vi "main.vi"() -> ()   [LabVIEW 2017]
uses:
  <vilib>/Platform/TimedLoop/XDataNode/timing_clust.ctl
  <vilib>/Platform/TimedLoop/XDataNode/nitl_modes.ctl
  <vilib>/Platform/TimedLoop/XDataNode/wakeup.ctl
  <vilib>/Instr/_visa.llb/VISA Configure Serial Port (Instr).vi
  <vilib>/Platform/TimedLoop/XDataNode/XDataNode.xnode
  <vilib>/Platform/TimedLoop/XDataNode/XDNodeRunTimeDep.lvlib
panel:
  out "TX":dbl
  out "RX":dbl
  in  "连接":bool
  out "串口状态":bool
  in  "波特率":u16(ring) items=["9600", "115200"]
  in  "端口":string(combo)
  in  "界面切换":enum32{"选项卡 1", "调试助手"}(tab)
  in  "清空波形":bool
  out "DA1计算值":dbl
  out "DA0计算值":dbl
  in  "清空曲线":bool
  in  "持续时间":string
  in  "系统时间":string
  in  "发送波形":bool
  out "波形图":dbl[](graph)
  in  "波形选择":enum32{"斜坡", "正弦", "PWM波", "直流", "抛物线", ""}(tab)
  out "斜率k":dbl format="%#.2g"
  in  "通道D":enum16{"DA0", "DA1", "DA01", ""}(ring) caption="通道"
  in  "截距":dbl(slide) min=-5.0 max=5.0 step=0.01 scale=-4.0..4.0
  in  "斜率角":dbl(slide) step=0.01 scale=0.0..180.0
  in  "极值":dbl(slide) min=-5.0 max=5.0 step=0.01 scale=-4.0..4.0
  out "正弦频率":dbl caption="频率 f" format="%#.2g"
  in  "偏距":dbl(slide) min=-5.0 max=5.0 step=0.01 scale=-4.0..4.0
  in  "初相":dbl(slide) min=-6.5 max=6.5 step=0.01 scale=-7.0..7.0
  in  "振幅":dbl(slide) min=0.0 max=5.0 step=0.01 scale=0.0..4.0
  in  "正弦角频率":dbl(slide) caption="角频率" min=0.0 max=100.0 step=0.01 scale=0.0..65.0
  in  "通道S":enum16{"DA0", "DA1", "DA01", ""}(ring) caption="通道"
  in  "通道P":enum16{"DA0", "DA1", "DA01", ""}(ring) caption="通道"
  in  "占空比":dbl(slide) min=0.0 max=1.0 step=0.01 scale=0.0..1.0
  in  "PWM波频率":dbl(slide) caption="频率" min=0.0 max=100.0 step=0.01 scale=0.0..10.0
  in  "低电压":dbl(slide) min=-5.0 max=5.0 step=0.01 scale=-4.0..4.0
  in  "高电压":dbl(slide) min=-5.0 max=5.0 step=0.01 scale=-4.0..4.0
  in  "DA0":dbl(slide) min=-5.0 max=5.0 step=0.01 scale=-4.0..4.0
  in  "DA1":dbl(slide) min=-5.0 max=5.0 step=0.01 scale=-4.0..4.0
  in  "板子选择":bool
  in  "换行":bool
  in  "发送区":string
  in  "send":bool
  in  "清空计数":bool
  in  "清空接收区":bool
  out "接收区":string
  # "y=kt+b"
  # "y=Asin(ωt+φ)+k"
  # "此页面无需点击“发送波形”按钮"
  # "y=k/(a*t+b)"
  # "y=kln(a)+b"
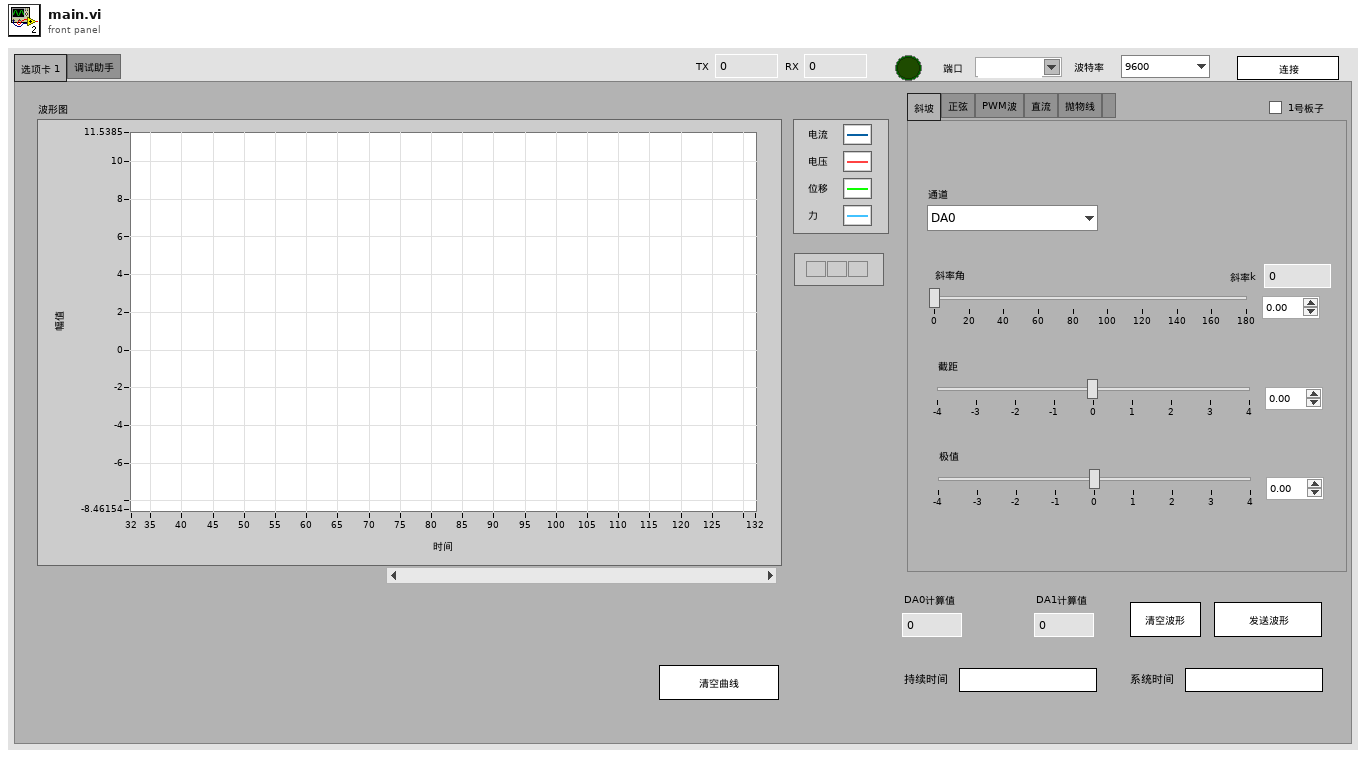
[diagram p1: front panel]
types:
  T1 = typedef "XDNodeRunTimeDep.lvlib/timing_clust.ctl" = cluster{"Expected End [f-1]":u64, "Actual End [f-1]":u64, "Finished Late? [f-1]":bool, "Expected End [i-1]":u64, "Actual End [i-1]":u64, "Finished Late? [i-1]":bool, "Expected Start [i]":u64, "Actual Start [i]":u64, "Expected Start [f]":u64, "Actual Start [f]":u64, "Source Name":string, "Structure Name":string, "Period":i64, "Deadline":i64, "Offset":i64, "Start":i64, "Priority":i32, "Timeout":i32, "Mode":T2, "Wakeup Reason":T3, "Error":errorcluster, "Source Type":string, "Secondary Source Type":string, "Global End Time":u64, "Global Start Time":u64, "Frame Duration":u64, "Iteration Duration":u64, "Assigned CPU":i32, "I/O Scan Engine Mode":u32}
  T2 = typedef "XDNodeRunTimeDep.lvlib/nitl_modes.ctl" = enum32{"No Change", "Process missed periods, maintain original phase", "Discard missed periods, maintain original phase", "Process missed periods, ignore original phase", "Discard missed periods, ignore original phase"}
  T3 = typedef "XDNodeRunTimeDep.lvlib/wakeup.ctl" = enum32{"Normal", "Aborted", "Asynchronous wakeup", "Timing source error", "Timed loop error", "Timeout"}
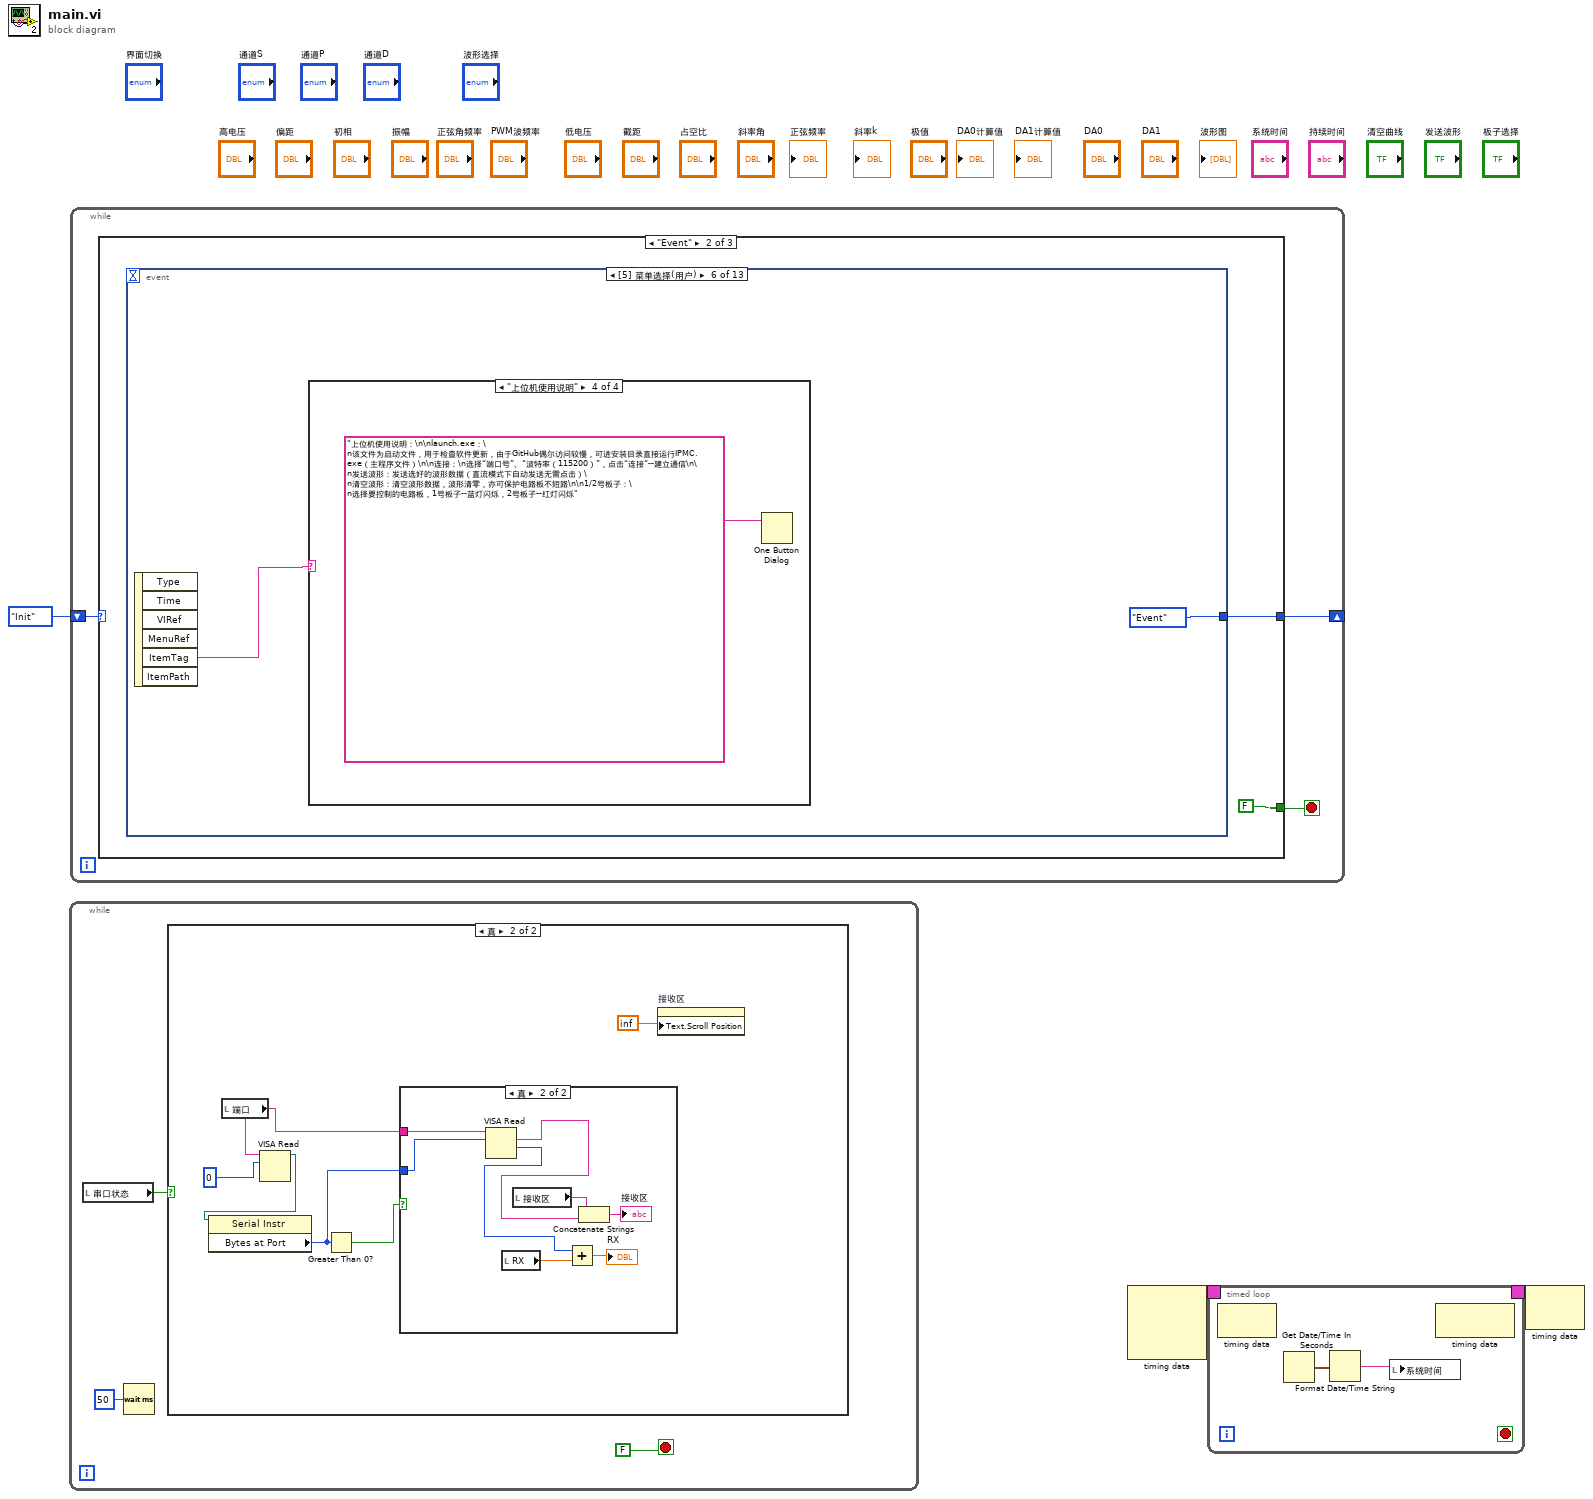
[diagram p0: block diagram]
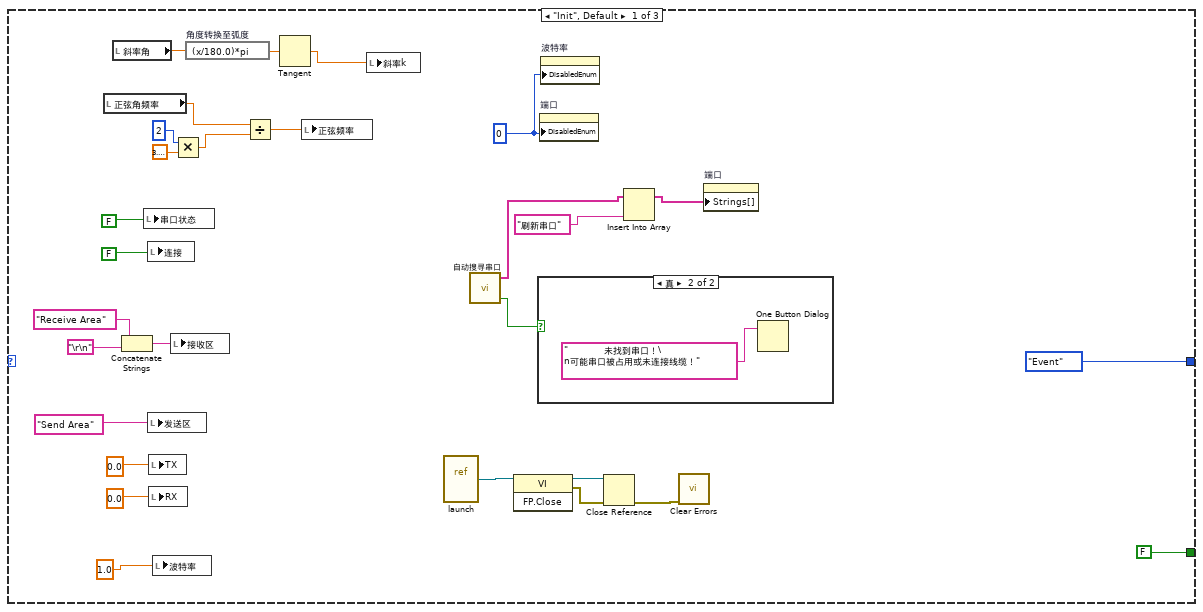
[diagram p4: hidden frame]
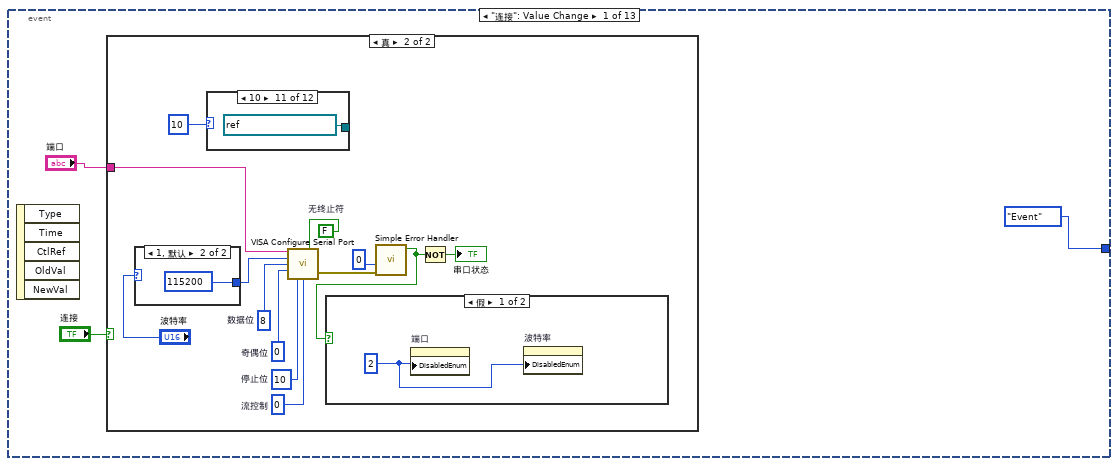
[diagram p6: hidden frame]
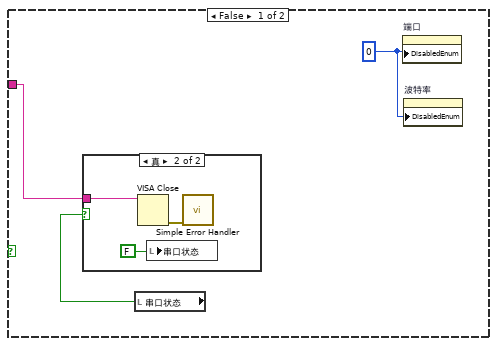
[diagram p7: hidden frame]
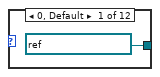
[diagram p9: hidden frame]
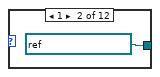
[diagram p10: hidden frame]
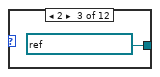
[diagram p11: hidden frame]
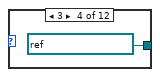
[diagram p12: hidden frame]
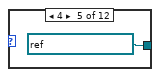
[diagram p13: hidden frame]
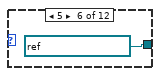
[diagram p14: hidden frame]
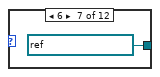
[diagram p15: hidden frame]
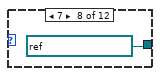
[diagram p16: hidden frame]
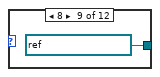
[diagram p17: hidden frame]
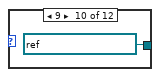
[diagram p18: hidden frame]
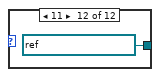
[diagram p19: hidden frame]
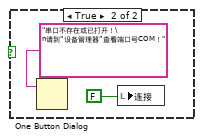
[diagram p20: hidden frame]
diagram:
  n1 = while {
    stop <- FALSE stop-if-true
    n2 = local read "串口状态"() -> (w6:bool)
    n3 = Wait (ms)(milliseconds to wait=u32 50 ("等待时间（毫秒）")) -> ()  [unwired: 1 out]
    n4 = case shown="真" w6 {
      frame False {
      }
      frame True {
        n5 = local read "端口"() -> (w10:string)
        n6 = VISA Read(VISA resource name=w10, byte count=0) -> (VISA resource name out=w9:refnum<visa-resource-name>)  [unwired: 1 in, 3 out]
        n7 = property class="Serial Instr"(reference=w9) -> ("Bytes at Port"=w7:u32)  [unwired: 1 in, 2 out]
        n8 = Greater Than 0?(x=w7) -> (x > 0?=w8:bool)
        n9 = case shown="真" w8 {
          tunnel: w10 -> [_ w14]
          tunnel: w7 -> [_ w13]
          frame False {
          }
          frame True {
            n10 = VISA Read(VISA resource name=w14, byte count=w13) -> (read buffer=w20:string, return count=w15:u32)  [unwired: 1 in, 2 out]
            n11 = local read "RX"() -> (w17:dbl)
            n12 = local read "接收区"() -> (w18:string)
            n13 = Add(x=w15, y=w17) -> (x+y=→"RX":dbl)
            n14 = Concatenate Strings(w18, w20) -> (→"接收区":string)
          }
        }
        n15 = property on="接收区" class="Str"("Text.Scroll Position"=inf) -> ()  [unwired: 2 in, 2 out]
      }
    }
  }
  n16 = while {
    shift-right: [w22] -> _
    shift-left: enum16{"Init", "Event", "Exit"}."Init" -> [w23]
    stop <- w21 stop-if-true
    n17 = case shown="\"Event\"" w23 {
      tunnel: [FALSE FALSE TRUE] -> w21
      tunnel: [enum16{"Init", "Event", "Exit"}."Event" w53 enum16{"Init", "Event", "Exit"}."Exit"] -> w22
      frame "Init", Default {
        w32 = 0
        n18 = local read "正弦角频率"() -> (w39:dbl)
        n19 = local read "斜率角"() -> (w43:dbl)
        n20 = Concatenate Strings("Receive Area", "\r\n") -> (w33:string)
        n21 = local write "串口状态"(FALSE) -> ()
        n22 = local write "连接"(FALSE) -> ()
        n23 = local write "发送区"("Send Area" ("发送区")) -> ()
        n24 = local write "TX"(0.0 ("TX")) -> ()
        n25 = local write "RX"(0.0 ("RX")) -> ()
        n26 = local write "波特率"(1.0 ("RX")) -> ()
        n27 = local write "接收区"(w33) -> ()
        n28 = Multiply(x=2, y=3.141592653589793) -> (x*y=w38:dbl)
        n29 = expression code="(x/180.0)*pi" "角度转换至弧度"(w43) -> (w44:dbl)
        n30 = Divide(x=w39, y=w38) -> (x/y=w40:dbl)
        n31 = Tangent(1:w44) -> (0:w37:dbl)
        n32 = local write "正弦频率"(w40) -> ()
        n33 = local write "斜率k"(w37) -> ()
        n34 = vi-ref "launch.vi"() -> (w27:refnum<vi>)
        n35 = call "自动搜寻串口.vi"() -> ("找到的串口"=w30:string[], "有错误?"=w31:bool)  [unwired: 6 in, 1 out]
        n36 = invoke class="VI" method="FP.Close"(reference=w27) -> (reference out=w26:refnum<vi>, error out=w25:errorcluster)  [unwired: 2 in, 1 out]
        n37 = case shown="真" w31 {
          frame False {
          }
          frame True {
            n38 = One Button Dialog(message="            未找到串口！\n可能串口被占用或未连接线缆！") -> ()  [unwired: 1 in, 1 out]
          }
        }
        n39 = property on="端口" class="CmbBox"("DisabledEnum"=w32) -> ()  [unwired: 2 in, 2 out]
        n40 = property on="波特率" class="Ring (严格)"("DisabledEnum"=w32) -> ()  [unwired: 2 in, 2 out]
        n41 = Close Reference(reference=w26, error in (no error)=w25) -> (error out=w24:errorcluster)
        n42 = Insert Into Array(array=w30, new element="刷新串口") -> (w28:string[])  [unwired: 1 in]
        n43 = call <vilib>:"Clear Errors.vi"("error in (no error)"=w24) -> ()  [unwired: 5 in, 2 out]
        n44 = property on="端口" class="CmbBox"("Strings[]"=w28) -> ()  [unwired: 2 in, 2 out]
      }
      frame "Event" {
        n45 = event shown="[5] 菜单选择(用户)" {
          selector: _ -> [_ _ _ _ _ _ _ _ _ _ _ _ _]
          dyn-events: _ -> [_ _ _ _ _ _ _ _ _ _ _ _ _]
          timeout: _ -> [_ _ _ _ _ _ _ _ _ _ _ _ _]
          tunnel: [enum16{"Init", "Event", "Exit"}."Event" _ enum16{"Init", "Event", "Exit"}."Event" enum16{"Init", "Event", "Exit"}."Event" enum16{"Init", "Event", "Exit"}."Event" enum16{"Init", "Event", "Exit"}."Event" enum16{"Init", "Event", "Exit"}."Event" enum16{"Init", "Event", "Exit"}."Event" enum16{"Init", "Event", "Exit"}."Event" enum16{"Init", "Event", "Exit"}."Event" enum16{"Init", "Event", "Exit"}."Event" enum16{"Init", "Event", "Exit"}."Event" enum16{"Init", "Event", "Exit"}."Event"] -> w53
          event "连接": Value Change {
            n46 = event-data() -> ()  [unwired: 1 in, 5 out]
            n47 = case shown="真" "连接" {
              tunnel: "端口" -> [w59 w64]
              frame False {
                w58 = 0
                n48 = local read "串口状态"() -> (w60:bool)
                n49 = case shown="真" w60 {
                  tunnel: w59 -> [_ w61]
                  frame False {
                  }
                  frame True {
                    n50 = VISA Close(VISA resource name=w61) -> (error out=w63:errorcluster)  [unwired: 1 in]
                    n51 = local write "串口状态"(FALSE) -> ()
                    n52 = call <vilib>:"Simple Error Handler.vi"("error in (no error)"=w63) -> ()  [unwired: 4 in, 5 out]
                  }
                }
                n53 = property on="端口" class="CmbBox"("DisabledEnum"=w58) -> ()  [unwired: 2 in, 2 out]
                n54 = property on="波特率" class="Ring (严格)"("DisabledEnum"=w58) -> ()  [unwired: 2 in, 2 out]
              }
              frame True {
                w67 = FALSE  # 无终止符
                w74 = u16 0  # 流控制
                w73 = u16 10  # 停止位
                w72 = u8 0  # 奇偶位
                w71 = u16 8  # 数据位
                n55 = case shown="1, 默认" "波特率" {
                  tunnel: [u32 9600 u32 115200] -> w70
                  frame 0 {
                  }
                  frame 1, Default {
                  }
                }
                n56 = case shown="10" 10 {
                  tunnel: [refnum<visa-resource-name> "ASRL1::INSTR" ("VISA resource name") refnum<visa-resource-name> "ASRL2::INSTR" ("VISA resource name") refnum<visa-resource-name> "ASRL3::INSTR" ("VISA resource name") refnum<visa-resource-name> "ASRL4::INSTR" ("VISA resource name") refnum<visa-resource-name> "ASRL5::INSTR" ("VISA resource name") refnum<visa-resource-name> "ASRL6::INSTR" ("VISA resource name") refnum<visa-resource-name> "ASRL7::INSTR" ("VISA resource name") refnum<visa-resource-name> "ASRL8::INSTR" ("VISA resource name") refnum<visa-resource-name> "ASRL9::INSTR" ("VISA resource name") refnum<visa-resource-name> "ASRL10::INSTR" ("VISA resource name") refnum<visa-resource-name> "ASRL11::INSTR" ("VISA resource name") refnum<visa-resource-name> "ASRL12::INSTR" ("VISA resource name")] -> _
                  frame 0, Default {
                  }
                  frame 1 {
                  }
                  frame 2 {
                  }
                  frame 3 {
                  }
                  frame 4 {
                  }
                  frame 5 {
                  }
                  frame 6 {
                  }
                  frame 7 {
                  }
                  frame 8 {
                  }
                  frame 9 {
                  }
                  frame 10 {
                  }
                  frame 11 {
                  }
                }
                n57 = call-poly "VISA Configure Serial Port"("VISA resource name"=w64, "Enable Termination\nChar (T)"=w67, "baud rate (9600)"=w70, "data bits (8)"=w71, "parity (0:none)"=w72, "stop bits (10: 1 bit)"=w73, "flow control (0:none)"=w74) -> ("error out"=w75:errorcluster)  [unwired: 7 in, 1 out]
                n58 = call <vilib>:"Simple Error Handler.vi"("type of dialog (OK msg:1)"=0, "error in (no error)"=w75) -> ("error?"=w68:bool)  [unwired: 3 in, 4 out]
                n59 = case shown="假" w68 {
                  frame False {
                    w89 = 2
                    n60 = property on="端口" class="CmbBox"("DisabledEnum"=w89) -> ()  [unwired: 2 in, 2 out]
                    n61 = property on="波特率" class="Ring (严格)"("DisabledEnum"=w89) -> ()  [unwired: 2 in, 2 out]
                  }
                  frame True {
                    n62 = One Button Dialog(message="串口不存在或已打开！\n请到“设备管理器”查看端口号COM！") -> ()  [unwired: 1 in, 1 out]
                    n63 = local write "连接"(FALSE) -> ()
                  }
                }
                n64 = Not(x=w68) -> (.not. x?=→"串口状态":bool)
              }
            }
          }
          event "端口": Value Change {
            n65 = event-data() -> ("NewVal"=w96:string)  [unwired: 1 in, 5 out]
            n66 = Equal?(x=w96, y="刷新串口") -> (x = y?=w94:bool)
            n67 = case shown="真" w94 {
              frame False {
              }
              frame True {
                n68 = call "自动搜寻串口.vi"() -> ("找到的串口"=w98:string[], "有错误?"=w100:bool)  [unwired: 6 in, 1 out]
                n69 = case shown="真" w100 {
                  frame False {
                  }
                  frame True {
                    n70 = One Button Dialog(message="            未找到串口！\n可能串口被占用或未连接线缆！") -> ()  [unwired: 1 in, 1 out]
                  }
                }
                n71 = Insert Into Array(array=w98, new element="刷新串口") -> (w97:string[])  [unwired: 1 in]
                n72 = property on="端口" class="CmbBox"("Strings[]"=w97) -> ()  [unwired: 2 in, 2 out]
              }
            }
          }
          event "send": Mouse Down {
            n73 = event-data() -> ()  [unwired: 1 in, 7 out]
            n74 = local read "串口状态"() -> (w103:bool)
            n75 = case shown="真" w103 {
              frame False {
              }
              frame True {
                n76 = local read "端口"() -> (w104:string)
                n77 = case shown="真" "换行" {
                  tunnel: [_ "\r"] -> w112
                  tunnel: [_ "\n"] -> w111
                  frame False {
                  }
                  frame True {
                  }
                }
                n78 = Concatenate Strings("发送区", w112, w111) -> (w108:string)
                n79 = local read "TX"() -> (w107:dbl)
                n80 = VISA Write(VISA resource name=w104, write buffer=w108) -> (return count=w105:u32)  [unwired: 1 in, 2 out]
                n81 = Add(x=w105, y=w107) -> (x+y=→"TX":dbl)
              }
            }
          }
          event "清空计数": Mouse Down {
            n82 = event-data() -> ()  [unwired: 1 in, 7 out]
            n83 = local write "RX"(0.0 ("RX")) -> ()
            n84 = local write "TX"(0.0 ("TX")) -> ()
          }
          event "清空接收区": Mouse Down {
            n85 = event-data() -> ()  [unwired: 1 in, 7 out]
            n86 = local write "接收区"("") -> ()
          }
          event Menu Selection (User) {
            n87 = event-data() -> ("ItemTag"=w120:string)  [unwired: 1 in, 5 out]
            n88 = case shown="\"上位机使用说明\"" w120 {
              frame "关于", Default {
                n89 = One Button Dialog(message="By IBSS, NUAA, YYH" ("Message")) -> ()  [unwired: 1 in, 1 out]
              }
              frame "数据协议" {
                n90 = call <vilib>:"Application Directory.vi"() -> ("Application Directory"=w126:path)
                n91 = call <vilib>:"System Exec.vi"("run minimized? (F)"=TRUE, "wait until completion? (T)"=FALSE, "working directory"=w126, "command line"="cmd /c start protocol.xlsx") -> ("error out"=w127:errorcluster)  [unwired: 4 in, 3 out]
                n92 = call <vilib>:"Simple Error Handler.vi"("error in (no error)"=w127) -> ()  [unwired: 4 in, 5 out]
              }
              frame "电路板使用说明" {
                n93 = One Button Dialog(message="电路板使用说明：\n\n灯光：\n常亮灯：电源指示灯\n闪烁灯：慢闪--工作指示\n            快闪--错误指示\n            颜色--板子编号（蓝LED0、红LED1）\n\n按键：\nKEY键（边缘）：切换板子编号\nRESET键（中间）：系统复位\n\nUSB口：用于和电脑连接\n\nCAN口：用于多电路板连接，CANH连CANH，CANL连CANL，并保证闪烁的灯颜色不一致\n\n电话口（RS232）：用于和激光位移传感器KEYENCE LKGD500连接") -> ()  [unwired: 1 in, 1 out]
              }
              frame "上位机使用说明" {
                n94 = One Button Dialog(message="上位机使用说明：\n\nlaunch.exe：\n该文件为启动文件，用于检查软件更新，由于GitHub偶尔访问较慢，可进安装目录直接运行IPMC.exe（主程序文件）\n\n连接：\n选择“端口号”、“波特率（115200）”，点击“连接”--建立通信\n\n发送波形：发送选好的波形数据（直流模式下自动发送无需点击）\n清空波形：清空波形数据，波形清零，亦可保护电路板不短路\n\n1/2号板子：\n选择要控制的电路板，1号板子--蓝灯闪烁，2号板子--红灯闪烁") -> ()  [unwired: 1 in, 1 out]
              }
            }
          }
          event "清空波形": Mouse Up {
            w132 = 3  # 类型强制直流
            w138 = 2  # 通道
            w140 = 170
            n95 = event-data() -> ()  [unwired: 1 in, 8 out]
            n96 = local read "板子选择"() -> (w131:bool)
            n97 = Boolean To (0,1)(Boolean=w131) -> (0, 1=w130:i16)
            n98 = call "浮点转字节数组.vi"("输入"=0.0) -> ("数组，高字节在前"=w134:u8[])  [unwired: 3 in, 4 out]
            n99 = Build Array (concatenate)(w140, w140, w130, w138, w132, w134, w134, 0) -> (w139:i32[])
            n100 = Byte Array To String(unsigned byte array=w139) -> (string=w136:string)
            n101 = local write "发送区"(w136) -> ()
            n102 = local read "串口状态"() -> (w135:bool)
            n103 = case shown="真" w135 {
              tunnel: w136 -> [_ w144]
              frame False {
                n104 = One Button Dialog(message="未连接平台！") -> ()  [unwired: 1 in, 1 out]
              }
              frame True {
                n105 = local read "端口"() -> (w143:string)
                n106 = Concatenate Strings(w144, "\r\n") -> (w149:string)
                n107 = local read "TX"() -> (w147:dbl)
                n108 = VISA Write(VISA resource name=w143, write buffer=w149) -> (return count=w148:u32)  [unwired: 1 in, 2 out]
                n109 = Add(x=w148, y=w147) -> (x+y=w145:dbl)
                n110 = local write "TX"(w145) -> ()
              }
            }
          }
          event "发送波形": Mouse Up {
            n111 = event-data() -> ()  [unwired: 1 in, 8 out]
            n112 = local read "板子选择"() -> (w151:bool)
            n113 = local read "波形选择"() -> (w155:enum32{"斜坡", "正弦", "PWM波", "直流", "抛物线", ""})
            n114 = Boolean To (0,1)(Boolean=w151) -> (0, 1=w150:i16)
            n115 = case shown="\"斜坡\", 默认" w155 {
              selector: w155 -> [w165 w178 w193 _]
              tunnel: [w172 w181 w196 "\r\n"] -> w153
              tunnel: w150 -> [w164 w177 w192 _]
              frame "斜坡", Default {
                w176 = 170
                n116 = local read "通道D"() -> (w166:enum16{"DA0", "DA1", "DA01", ""})
                n117 = local read "斜率k"() -> (w171:dbl)
                n118 = local read "极值"() -> (w169:dbl)
                n119 = local read "截距"() -> (w174:dbl)
                n120 = call "浮点转字节数组.vi"("输入"=w169) -> ("数组，高字节在前"=w167:u8[])  [unwired: 3 in, 4 out]
                n121 = call "浮点转字节数组.vi"("输入"=w171) -> ("数组，高字节在前"=w175:u8[])  [unwired: 3 in, 4 out]
                n122 = call "浮点转字节数组.vi"("输入"=w174) -> ("数组，高字节在前"=w173:u8[])  [unwired: 3 in, 4 out]
                n123 = Build Array (concatenate)(w176, w176, w164, w166, w165, w175, w173, w167, 0) -> (w170:u32[])
                n124 = Byte Array To String(unsigned byte array=w170) -> (string=w172:string)
                n125 = local write "发送区"(w172) -> ()
              }
              frame "正弦" {
                w191 = 170
                n126 = local read "通道S"() -> (w179:enum16{"DA0", "DA1", "DA01", ""})
                n127 = local read "正弦角频率"() -> (w188:dbl)
                n128 = local read "初相"() -> (w187:dbl)
                n129 = local read "偏距"() -> (w183:dbl)
                n130 = local read "振幅"() -> (w190:dbl)
                n131 = call "浮点转字节数组.vi"("输入"=w190) -> ("数组，高字节在前"=w189:u8[])  [unwired: 3 in, 4 out]
                n132 = call "浮点转字节数组.vi"("输入"=w188) -> ("数组，高字节在前"=w186:u8[])  [unwired: 3 in, 4 out]
                n133 = call "浮点转字节数组.vi"("输入"=w187) -> ("数组，高字节在前"=w185:u8[])  [unwired: 3 in, 4 out]
                n134 = call "浮点转字节数组.vi"("输入"=w183) -> ("数组，高字节在前"=w184:u8[])  [unwired: 3 in, 4 out]
                n135 = Build Array (concatenate)(w191, w191, w177, w179, w178, w189, w186, w185, w184, 0) -> (w180:u32[])
                n136 = Byte Array To String(unsigned byte array=w180) -> (string=w181:string)
                n137 = local write "发送区"(w181) -> ()
              }
              frame "PWM波" {
                w206 = 170
                n138 = local read "通道P"() -> (w194:enum16{"DA0", "DA1", "DA01", ""})
                n139 = local read "PWM波频率"() -> (w201:dbl)
                n140 = local read "占空比"() -> (w199:dbl)
                n141 = local read "高电压"() -> (w205:dbl)
                n142 = local read "低电压"() -> (w203:dbl)
                n143 = call "浮点转字节数组.vi"("输入"=w205) -> ("数组，高字节在前"=w204:u8[])  [unwired: 3 in, 4 out]
                n144 = call "浮点转字节数组.vi"("输入"=w203) -> ("数组，高字节在前"=w202:u8[])  [unwired: 3 in, 4 out]
                n145 = call "浮点转字节数组.vi"("输入"=w201) -> ("数组，高字节在前"=w200:u8[])  [unwired: 3 in, 4 out]
                n146 = call "浮点转字节数组.vi"("输入"=w199) -> ("数组，高字节在前"=w198:u8[])  [unwired: 3 in, 4 out]
                n147 = Build Array (concatenate)(w206, w206, w192, w194, w193, w204, w202, w200, w198, 0) -> (w195:u32[])
                n148 = Byte Array To String(unsigned byte array=w195) -> (string=w196:string)
                n149 = local write "发送区"(w196) -> ()
              }
              frame "直流" {
              }
            }
            n150 = local read "串口状态"() -> (w154:bool)
            n151 = case shown="真" w154 {
              tunnel: w153 -> [_ w158]
              frame False {
                n152 = One Button Dialog(message="未连接平台！") -> ()  [unwired: 1 in, 1 out]
              }
              frame True {
                n153 = local read "端口"() -> (w157:string)
                n154 = Concatenate Strings(w158, "\r\n") -> (w163:string)
                n155 = local read "TX"() -> (w161:dbl)
                n156 = VISA Write(VISA resource name=w157, write buffer=w163) -> (return count=w162:u32)  [unwired: 1 in, 2 out]
                n157 = Add(x=w162, y=w161) -> (x+y=w159:dbl)
                n158 = local write "TX"(w159) -> ()
              }
            }
          }
          event "DA0": Value Change {
            w211 = 0  # 通道
            w221 = 170
            n159 = event-data() -> ()  [unwired: 1 in, 6 out]
            n160 = local read "板子选择"() -> (w209:bool)
            n161 = local read "波形选择"() -> (w210:enum32{"斜坡", "正弦", "PWM波", "直流", "抛物线", ""})
            n162 = Boolean To (0,1)(Boolean=w209) -> (0, 1=w208:i16)
            n163 = local read "DA0"() -> (w220:dbl)
            n164 = local read "DA1"() -> (w219:dbl)
            n165 = call "浮点转字节数组.vi"("输入"=w220) -> ("数组，高字节在前"=w218:u8[])  [unwired: 3 in, 4 out]
            n166 = call "浮点转字节数组.vi"("输入"=w219) -> ("数组，高字节在前"=w217:u8[])  [unwired: 3 in, 4 out]
            n167 = Build Array (concatenate)(w221, w221, w208, w211, w210, w218, w217, 0) -> (w215:u32[])
            n168 = Byte Array To String(unsigned byte array=w215) -> (string=w213:string)
            n169 = local write "发送区"(w213) -> ()
            n170 = local read "串口状态"() -> (w214:bool)
            n171 = case shown="真" w214 {
              tunnel: w213 -> [_ w224]
              frame False {
                n172 = One Button Dialog(message="未连接平台！") -> ()  [unwired: 1 in, 1 out]
              }
              frame True {
                n173 = local read "端口"() -> (w223:string)
                n174 = Concatenate Strings(w224, "\r\n") -> (w229:string)
                n175 = local read "TX"() -> (w227:dbl)
                n176 = VISA Write(VISA resource name=w223, write buffer=w229) -> (return count=w228:u32)  [unwired: 1 in, 2 out]
                n177 = Add(x=w228, y=w227) -> (x+y=w225:dbl)
                n178 = local write "TX"(w225) -> ()
              }
            }
          }
          event "DA1": Value Change {
            w233 = 1  # 通道
            w243 = 170
            n179 = event-data() -> ()  [unwired: 1 in, 6 out]
            n180 = local read "板子选择"() -> (w231:bool)
            n181 = local read "波形选择"() -> (w232:enum32{"斜坡", "正弦", "PWM波", "直流", "抛物线", ""})
            n182 = local read "DA0"() -> (w235:dbl)
            n183 = local read "DA1"() -> (w236:dbl)
            n184 = Boolean To (0,1)(Boolean=w231) -> (0, 1=w230:i16)
            n185 = call "浮点转字节数组.vi"("输入"=w235) -> ("数组，高字节在前"=w242:u8[])  [unwired: 3 in, 4 out]
            n186 = call "浮点转字节数组.vi"("输入"=w236) -> ("数组，高字节在前"=w241:u8[])  [unwired: 3 in, 4 out]
            n187 = Build Array (concatenate)(w243, w243, w230, w233, w232, w242, w241, 0) -> (w239:u32[])
            n188 = Byte Array To String(unsigned byte array=w239) -> (string=w238:string)
            n189 = local read "串口状态"() -> (w234:bool)
            n190 = case shown="真" w234 {
              tunnel: w238 -> [_ w246]
              frame False {
                n191 = One Button Dialog(message="未连接平台！") -> ()  [unwired: 1 in, 1 out]
              }
              frame True {
                n192 = local read "端口"() -> (w245:string)
                n193 = Concatenate Strings(w246, "\r\n") -> (w251:string)
                n194 = local read "TX"() -> (w249:dbl)
                n195 = VISA Write(VISA resource name=w245, write buffer=w251) -> (return count=w250:u32)  [unwired: 1 in, 2 out]
                n196 = Add(x=w250, y=w249) -> (x+y=w247:dbl)
                n197 = local write "TX"(w247) -> ()
              }
            }
          }
          event "斜率角": Value Change {
            n198 = event-data() -> ("NewVal"=w255:dbl)  [unwired: 1 in, 5 out]
            n199 = expression code="(x/180.0)*pi" "角度转换至弧度"(w255) -> (w254:dbl)
            n200 = Tangent(1:w254) -> (0:w252:dbl)
            n201 = local write "斜率k"(w252) -> ()
          }
          event "正弦角频率": Value Change {
            n202 = event-data() -> ("NewVal"=w258:dbl)  [unwired: 1 in, 5 out]
            n203 = Multiply(x=2, y=3.141592653589793) -> (x*y=w257:dbl)
            n204 = Divide(x=w258, y=w257) -> (x/y=w256:dbl)
            n205 = local write "正弦频率"(w256) -> ()
          }
          event "高电压", "低电压": Value Change {
            n206 = event-data() -> ()  [unwired: 1 in, 6 out]
            n207 = local read "高电压"() -> (w264:dbl)
            n208 = local read "低电压"() -> (w263:dbl)
            n209 = Greater Or Equal?(x=w264, y=w263) -> (x >= y?=w265:bool)
            n210 = case shown="假" w265 {
              tunnel: w263 -> [w266 _]
              frame False {
                n211 = local write "高电压"(w266) -> ()
              }
              frame True {
              }
            }
          }
        }
      }
      frame "Exit" {
      }
    }
  }
  n212 = node-c288() -> (w2:T1)  [unwired: 3 in]
  n213 = timed-loop {
    timing: w2 -> [_]
    timing-out: [_] -> w1
    stop <- _ stop-if-true
    n214 = node-c288() -> ()  [unwired: 1 in, 1 out]
    n215 = Get Date/Time In Seconds() -> (seconds since 1Jan1904=w270:timestamp)
    n216 = Format Date/Time String(seconds (now)=w270) -> (date/time string=w269:string)  [unwired: 2 in]
    n217 = local write "系统时间"(w269) -> ()
    n218 = node-c288() -> ()  [unwired: 1 in, 1 out]
  }
  n219 = node-c288(w1) -> ()  [unwired: 1 out]
